vi "KepcoDCPwr Close.vi"(0 "VISA Session":refnum<visa-resource-name>, 11 "error in (no error)":errorcluster {"code" format="%.0x"}) -> (15 "error out":errorcluster {"code" format="%.0x"})   [LabVIEW 2013]
doc: "This VI performs the following operations:\n\n- Closes the instrument I/O session.\n\n- Destroys the instrument driver session and all of its properties.\n\n- Deallocates any memory resources the driver uses.\n\nNotes:\n\n(1) You must unlock the session before calling KepcoDCPwr Close.vi.\n\n(2) After calling KepcoDCPwr Close.vi, you cannot use the instrument driver again until you call KepcoDCPwr Initialize.vi or KepcoDCPwr Initialize With Options.vi."
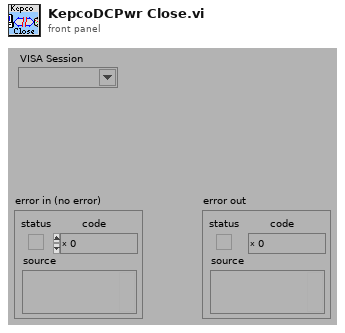
[diagram p1: front panel]
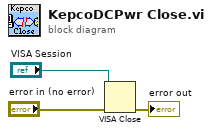
[diagram p0: block diagram]
diagram:
  n1 = VISA Close(VISA resource name="VISA Session", error in (no error)="error in (no error)") -> (error out=→"error out":errorcluster)
